vi "Create TestComplete Reader.vi"(8 "error in (no error)":errorcluster) -> (0 "error out":errorcluster, 3 "reader endpoint":refnum<k21>)   [LabVIEW 2019]
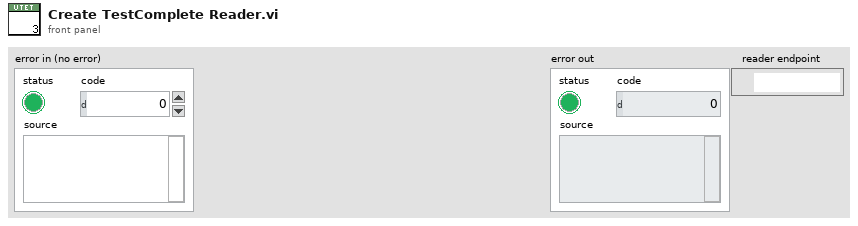
[diagram p1: front panel]
types:
  T1 = cluster{"Socket":i32, "SerialNumber":string, "TestResult":string}
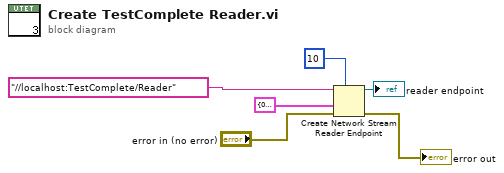
[diagram p0: block diagram]
diagram:
  n1 = Create Network Stream Reader Endpoint(7:10 ("reader buffer size"), 8:"error in (no error)", 9:T1 {"Socket"=0, "SerialNumber"="", "TestResult"=""}, 11:"//localhost:TestComplete/Reader" ("reader name")) -> (0:→"error out":errorcluster, 3:→"reader endpoint":refnum<k21>)  [unwired: 3 in]
